vi "Write I64.vi"(8 "error in (no error)":errorcluster, 9 "Timeout (ms)":i32, 10 "Data":i64, 11 "CIFTag in":refnum<class "CIFTagI64.lvclass">) -> (0 "error out":errorcluster, 1 "timed out?":bool, 3 "CIFTag out":refnum<class "CIFTagI64.lvclass">)   [LabVIEW 2021, in "CIFTagI64.lvclass"]
uses:
  CIFTagI64.lvclass
  CIFTagI64.lvclass/CIFTagI64.ctl
  e6e5dc56-0fe0-434b-816e-55c2e61471c2.vi
  CIFTag/CIFTag.lvclass
  D:/dev/CIF-LVCore/src/Channels/CIFTag/CIFTag/CIFTag.lvclass
  D:/dev/CIF-LVCore/src/CIFUtilities/CIFChannels/CIFChannels.lvclass
  D:/dev/CIF-LVCore/src/Channels/CIFTag/I64/CIFTagI64.lvclass
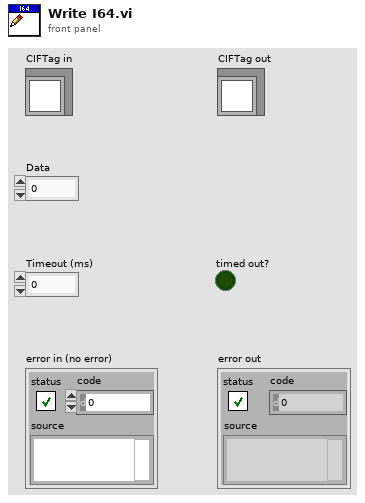
[diagram p1: front panel]
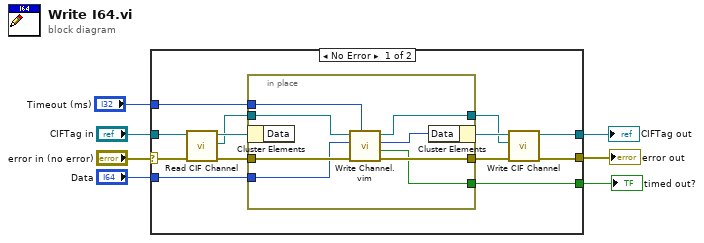
[diagram p0: block diagram]
diagram:
  n1 = case shown="No Error" "error in (no error)" {
    selector: "error in (no error)" -> [w17 w30]
    tunnel: [w11 w30] -> w6
    tunnel: [w13 w29] -> w4
    tunnel: "CIFTag in" -> [w18 w29]
    tunnel: "Data" -> [w20 _]
    tunnel: [w19 _] -> w2
    tunnel: "Timeout (ms)" -> [w8 _]
    frame No Error {
      n2 = call "Read CIF Channel.vi"("error in (no error)"=w17, "CIFTag in"=w18) -> ("error out"=w15:errorcluster, "CIF Channel"=w10:refnum<k21>, "CIFTag out"=w16:refnum<class "CIFTagI64.lvclass">)  [unwired: 7 in]
      n3 = in-place {
        in-place-border: w15 -> [w28]
        in-place-border: [w27] -> w12
        in-place-border: w20 -> [w25]
        in-place-border: [w26] -> w19
        in-place-border: w10 -> [w23]
        in-place-border: [w22] -> w9
        in-place-border: w8 -> [w21]
        n4 = in-place-cluster #1(w16) -> ()  [unwired: 1 out]
        n5 = call "Write Channel.vim"("Timeout (ms)"=w21, "error in"=w28, "Data in"=w25, "CIF Channel in"=w23) -> ("error out"=w27:errorcluster, "Timed out?"=w26:bool, "Data out"=w24:i64, "CIF Channel out"=w22:refnum<k21>)  [unwired: 4 in]
        n6 = in-place-cluster #1("Data"=w24) -> (w14:refnum<class "CIFTagI64.lvclass">)
      }
      n7 = call "Write CIF Channel.vi"("error in (no error)"=w12, "CIF Channel"=w9, "CIFTag in"=w14) -> ("error out"=w11:errorcluster, "CIFTag out"=w13:refnum<class "CIFTagI64.lvclass">)  [unwired: 7 in]
    }
    frame Error {
    }
  }
  "error out" <- w6
  "CIFTag out" <- w4
  "timed out?" <- w2
